vi "OAT Even Angle Signal Sample Rate Conversion (N Channels).vi"(0 "even-angle signals":cluster{"r0":dbl, "dr":dbl, "Y":dbl[]}[](array[cluster]) {"r0" format="%.2p"; "dr" format="%.2p"; "Y" format="%.2f"}, 2 "reset? (F)":bool, 5 "even-angle channel info":T2[](array[typedef]) {"channel info"."pregain" format="%.2f"; "channel info"."weighting filter" items=["Linear", "A-weighting", "B-weighting", "C-weighting", "ITU-R 468-4", "Dolby", "CCITT", "C-message", "Wb", "Wc", "Wd", "We", "Wf", "Wh", "Wj", "Wk", "Wm", "AES17 20 kHz lowpass", "AES17 40 kHz lowpass", "AES17 20 kHz highpass", "AES17 40 kHz highpass"]; "channel info"."dB reference" format="%^.1e"; "channel info"."engineering units" items=["custom..."=0, "V"=1, "A"=21, "C"=30, "pC"=31, "s"=32, "-"=29, "Pa"=2, "N"=20, "g"=3, "m/s^2"=4, "m/s"=5, "m"=6, "mm/s"=12, "mm"=13, "micron/s"=14, "micron"=15, "in/s^2"=7, "in/s"=8, "in"=9, "mil/s"=10, "mil"=11, "rad/s^2"=16, "rad/s"=17, "rad"=18, "deg/s^2"=26, "deg/s"=27, "deg"=28, "RPM"=22, "cycle/s^2"=23, "Hz"=24, "cycle"=25, "strain"=19]; "channel info"."sensor sensitivity" format="%#_5f"}, 7 "even-angle position info":T1, 9 "new dr":dbl=1.0 format="%.2p", 11 "error in (no error)":errorcluster, 12 "interpolation mode":u16(ring)=1 items=["coerce", "linear", "spline", "FIR filter"], 13 "FIR filter specifications":T6={"alias rejection [dB]"=120.0, "normalized bandwidth"=0.4536} {"normalized bandwidth" format="%.4f"; "alias rejection [dB]" format="%.2f"}) -> (4 "even-angle signals out":cluster{"r0":dbl, "dr":dbl, "Y":dbl[]}[](array[cluster]) {"r0" format="%.2p"; "dr" format="%.2p"; "Y" format="%.2f"}, 6 "even-angle channel info out":T2[](array[typedef]) {"channel info"."pregain" format="%.2f"; "channel info"."weighting filter" items=["Linear", "A-weighting", "B-weighting", "C-weighting", "ITU-R 468-4", "Dolby", "CCITT", "C-message", "Wb", "Wc", "Wd", "We", "Wf", "Wh", "Wj", "Wk", "Wm", "AES17 20 kHz lowpass", "AES17 40 kHz lowpass", "AES17 20 kHz highpass", "AES17 40 kHz highpass"]; "channel info"."dB reference" format="%^.1e"; "channel info"."engineering units" items=["custom..."=0, "V"=1, "A"=21, "C"=30, "pC"=31, "s"=32, "-"=29, "Pa"=2, "N"=20, "g"=3, "m/s^2"=4, "m/s"=5, "m"=6, "mm/s"=12, "mm"=13, "micron/s"=14, "micron"=15, "in/s^2"=7, "in/s"=8, "in"=9, "mil/s"=10, "mil"=11, "rad/s^2"=16, "rad/s"=17, "rad"=18, "deg/s^2"=26, "deg/s"=27, "deg"=28, "RPM"=22, "cycle/s^2"=23, "Hz"=24, "cycle"=25, "strain"=19]; "channel info"."sensor sensitivity" format="%#_5f"}, 8 "even-angle position info out":T1, 15 "error out":errorcluster)   [LabVIEW 2017, in "SoundVib_OAUtility.lvlib"]
doc: "Converts the sample rate of the even-angle signal. Use this VI to specify a new revolution interval for sampling. Each instance of this VI maintains its own state; use the N waveforms instance of this VI to process an array of channels. Wire data to the <B>even-angle signal</B> input to determine the polymorphic instance to use or manually select the instance."
uses:
  <vilib>/addons/Sound and Vibration/Order Analysis/Utility/SoundVib_OAUtility.lvlib
  <vilib>/addons/Sound and Vibration/Order Analysis/Misc/OAT Position Info.ctl
  <vilib>/addons/_NISVFA/_Shared subVIs/Controls/svc_Resampled Channel Info.ctl
  <vilib>/addons/_NISVFA/_Shared subVIs/Controls/svc_Channel Info.ctl
  <vilib>/addons/_NISVFA/_Shared subVIs/Controls/svc_Engineering Units Text Ring.ctl
  <vilib>/addons/_NISVFA/_Shared subVIs/Controls/svc_Weighting Filter Text Ring.ctl
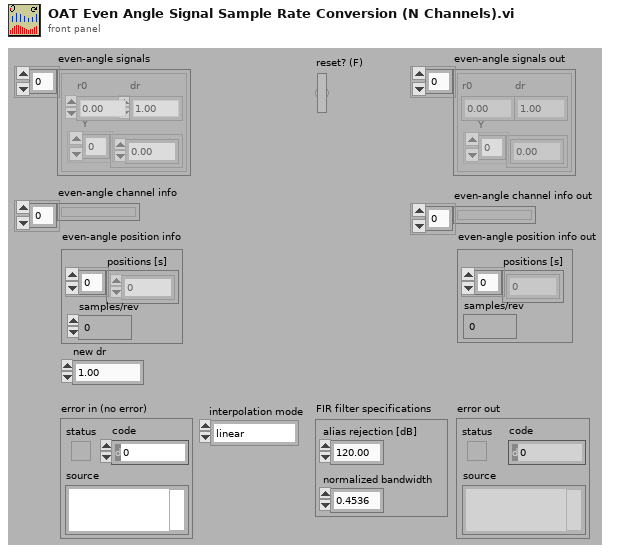
[diagram p1: front panel]
types:
  T1 = typedef "OAT Position Info.ctl" = cluster{"positions [s]":dbl[], "samples/rev":dbl}
  T2 = typedef "svc_Resampled Channel Info.ctl" = cluster{"channel name":string, "description":string, " channel info":T3}
  T3 = typedef "svc_Channel Info.ctl" = cluster{"sensor sensitivity":dbl, "engineering units":T4, "dB reference":dbl, "custom label":string, "weighting filter":T5, "pregain":dbl}
  T4 = typedef "svc_Engineering Units Text Ring.ctl" = u16
  T5 = typedef "svc_Weighting Filter Text Ring.ctl" = u16
  T6 = cluster{"alias rejection [dB]":dbl, "normalized bandwidth":dbl}
  T7 = cluster{"alias rejection (dB)":dbl, "normalized bandwidth":dbl}
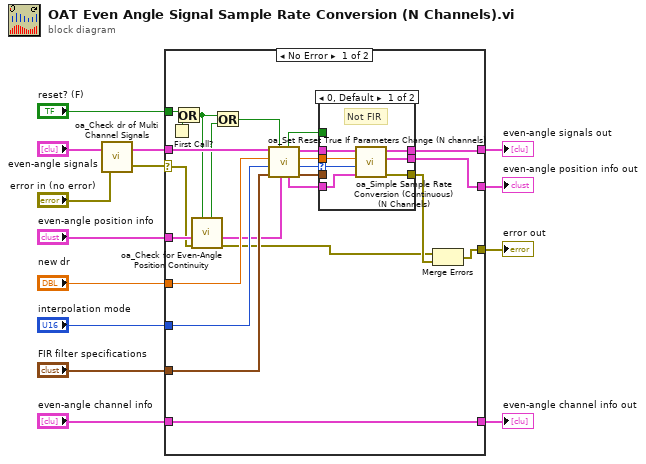
[diagram p0: block diagram]
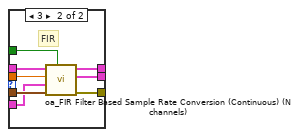
[diagram p2: hidden frame]
diagram:
  n1 = call <vilib>:"oa_Check dr of Multi Channel Signals.vi"("error in (no error)"="error in (no error)", "even angle signals in"="even-angle signals") -> ("error out"=w1:errorcluster, "even angle signals out"=w3:cluster{"r0":dbl, "dr":dbl, "Y":dbl[]}[])
  n2 = case shown="No Error" w1 {
    selector: w1 -> [w16 w55]
    tunnel: w3 -> [w38 w57]
    tunnel: "new dr" -> [w37 _]
    tunnel: "interpolation mode" -> [w36 _]
    tunnel: "FIR filter specifications" -> [w35 _]
    tunnel: [w25 w57] -> w5
    tunnel: [w22 w55] -> w11
    tunnel: "even-angle channel info" -> [w33 w56]
    tunnel: [w33 w56] -> w9
    tunnel: "even-angle position info" -> [w34 w54]
    tunnel: [w24 w54] -> w7
    tunnel: "reset? (F)" -> [w27 _]
    frame No Error {
      n3 = First Call?() -> (First Call?: T/F=w21:bool)
      n4 = Or(x=w27, y=w21) -> (x .or. y?=w19:bool)
      n5 = call <vilib>:"oa_Check for Even-Angle Position Continuity.vi"("reset in"=w19, "error in (no error)"=w16, "even-angle position info"=w34) -> ("error out"=w15:errorcluster, "even-angle position info dup"=w20:T1, "position not continuous"=w17:bool)  [unwired: 6 in]
      n6 = Or(x=w19, y=w17) -> (x .or. y?=w18:bool)
      n7 = call <vilib>:"oa_Set Reset True If Parameters Change (N channels).vi"("even angle position info"=w20, "reset? (T) in"=w18, "FIR filter specifications in"=w35, "interpolation mode in"=w36, "dr in"=w37, "even angle signals"=w38) -> ("FIR filter specifications out"=w29:T7, "interpolation mode out"=w32:u16, "dr out"=w30:dbl, "even angle signals out"=w31:cluster{"r0":dbl, "dr":dbl, "Y":dbl[]}[], "even angle position info out"=w28:T1, "reset? (T) out"=w26:bool)
      n8 = case shown="0, Default" w32 {
        selector: w32 -> [w44 _]
        tunnel: w31 -> [w43 w52]
        tunnel: w30 -> [w45 w51]
        tunnel: w29 -> [_ w53]
        tunnel: w28 -> [w42 w50]
        tunnel: w26 -> [_ w46]
        tunnel: [w41 w47] -> w25
        tunnel: [w40 w48] -> w24
        tunnel: [w39 w49] -> w23
        frame 0, Default {
          # "Not FIR"
          n9 = call <vilib>:"oa_Simple Sample Rate Conversion (Continuous) (N Channels).vi"("even angle position info"=w42, "interpolation mode"=w44, "dr"=w45, "even angle signals"=w43) -> ("error out"=w39:errorcluster, "out even angle position info"=w40:T1, "even angle signals out"=w41:cluster{"r0":dbl, "dr":dbl, "Y":dbl[]}[])  [unwired: 5 in]
        }
        frame 3 {
          # "FIR"
          n10 = call <vilib>:"oa_FIR Filter Based Sample Rate Conversion (Continuous) (N channels).vi"("reset? (T)"=w46, "FIR filter specifications"=w53, "even angle position info"=w50, "dr"=w51, "even angle signals"=w52) -> ("error out"=w49:errorcluster, "out even angle position info out"=w48:T1, "even angle signals out"=w47:cluster{"r0":dbl, "dr":dbl, "Y":dbl[]}[])  [unwired: 4 in]
        }
      }
      n11 = Merge Errors(w15, w23) -> (w22:errorcluster)
    }
    frame Error {
    }
  }
  "error out" <- w11
  "even-angle signals out" <- w5
  "even-angle channel info out" <- w9
  "even-angle position info out" <- w7
